vi "Configure Multipoint.vi"(8 "error in (no error)":errorcluster, 9 "Sample Count (1)":i32=1 format="%#.6g", 10 "Trigger Count (1)":i32=1 format="%#.6g", 11 "VISA resource name":refnum<visa-resource-name>) -> (0 "error out":errorcluster, 3 "VISA resource name out":refnum<visa-resource-name>)   [LabVIEW 2022 SP3, in "Agilent 34420.lvlib"]
doc: "Configures trigger count and sample count so you can take multipoint measurements.\n\n<B>Note:</B>\n\nUse this VI only with other low-level VIs. The high-level VIs automatically incorporate this functionality.\n\nWhen using low level <B>Initiate</B> and <B>Fetch Multiple Points</B> VI's the product of the <B>Sample Count</B> and <B>Trigger Count</B> can not exceed 1024 due to the limitation of the internal instrument buffer. When the instrument buffer is disabled via the <B>Configure Math</B> VI this restriction doesn't apply."
uses:
  Agilent 34420.lvlib
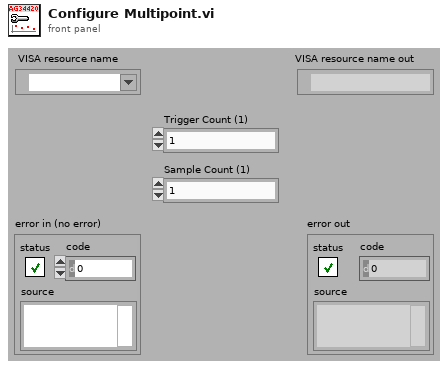
[diagram p1: front panel]
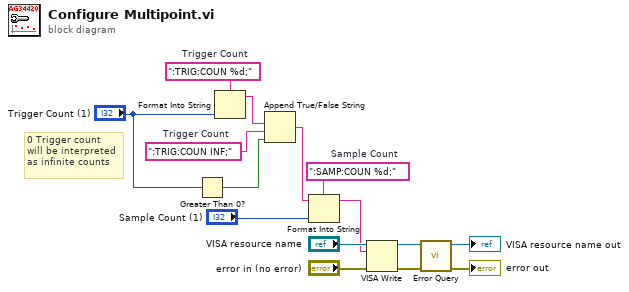
[diagram p0: block diagram]
diagram:
  w5 = ":TRIG:COUN INF;"  # Trigger Count
  w8 = ":SAMP:COUN %d;"  # Sample Count
  w9 = ":TRIG:COUN %d;"  # Trigger Count
  # "0 Trigger count\nwill be interpreted\nas infinite counts"
  n1 = Greater Than 0?(x="Trigger Count (1)") -> (x > 0?=w1:bool)
  n2 = Format Into String(format string=w9, "Trigger Count (1)") -> (resulting string=w4:string)  [unwired: 2 in, 1 out]
  n3 = Append True/False String(1:w1, 2:w5, 3:w4) -> (0:w3:string)  [unwired: 1 in]
  n4 = Format Into String(format string=w8, initial string=w3, "Sample Count (1)") -> (resulting string=w6:string)  [unwired: 1 in, 1 out]
  n5 = VISA Write(VISA resource name="VISA resource name", write buffer=w6, error in (no error)="error in (no error)") -> (VISA resource name out=w11:refnum<visa-resource-name>, error out=w10:errorcluster)  [unwired: 1 out]
  n6 = call "Error Query.vi"("error in (no error)"=w10, "VISA resource name"=w11) -> ("error out"=→"error out":errorcluster, "VISA resource name out"=→"VISA resource name out":refnum<visa-resource-name>)  [unwired: 6 in, 2 out]
